vi "Alle Rohdaten abholen.vi"(7 "automatisch":bool, 8 "error in (no error)":errorcluster caption="Fehler (Eingang, kein Fehler)", 10 "Temp. Messzelle G-nr.":i32, 11 "Gasindex":i32) -> (0 "error out":errorcluster caption="Fehler (Ausgang)", 3 "Gasindex out":i32)   [LabVIEW 2020, in "Linearisierung v2.lvlib"]
uses:
  Linearisierung v2.lvlib
  Messdaten/Aktionen FGV Messdaten.ctl
  Aktion FGV Rohmesswerte sammeln.ctl
  Seiten/FT-IR/Aktionen EVID-Codes.ctl
  Seiten/FT-IR/FGV FT-IR Aktionen.ctl
  Messdaten/Gewichtung (Stichprobe).ctl
  Messdaten/Messdaten.lvlib
  Seiten/FT-IR/FT-IR.lvlib
  Seiten/FT-IR/FGV FT-IR Gasliste Aktionen.ctl
  cRIO/PC/Kommunikation mit cRIO.lvlib
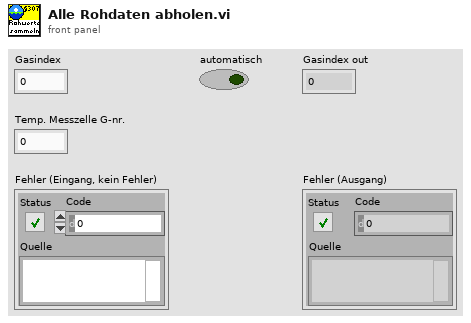
[diagram p1: front panel]
types:
  T1 = typedef "FT-IR.lvlib/FGV FT-IR Aktionen.ctl" = enum16{"lesen", "NOG setzen", "NOS setzen", "Initialisieren", "speichern", "ALLES setzen", "FT-IR Spektrum loggen", "Komm Stoppen", "Spektrum LogKonfig"}
  T2 = typedef "FT-IR.lvlib/Aktionen EVID-Codes.ctl" = enum16{"lesen", "setzen", "laden", "speichern", "1Hz/5Hz", "Smoothing", "Rolling Average"}
  T3 = typedef "Linearisierung v2.lvlib/Aktion FGV Rohmesswerte sammeln.ctl" = enum16{"lesen", "schreiben", "löschen", "Sollwert HovaCal"}
  T4 = typedef "Messdaten.lvlib/Aktionen FGV Messdaten.ctl" = enum16{"lesen", "schreiben", "löschen", "Mittelwerte", "Komponente"}
  T5 = typedef "FT-IR.lvlib/FGV FT-IR Gasliste Aktionen.ctl" = enum16{"lesen", "Gasliste FT-IR", "Gasliste ausgelesen", "laden", "speichern", "löschen"}
  T6 = typedef "String - Ausgabefeld.ctl" = string
  T7 = typedef "FT-IR.lvlib/1Hz-5Hz Geraet.ctl" = u16
  T8 = typedef "Verwaltung - cRIO.lvlib/Analog Eingaenge.ctl" = cluster{"AI0: Durchfluss FT-IR":sgl, "AI1: Druck Ausgang":sgl, "AI2: Umgebungsdruck":sgl, "AI3: Druck FT-IR":sgl, "AI4: Druck CalGas":sgl, "AI5: Reserve":sgl, "AI6: Reserve":sgl, "AI7: Reserve":sgl, "Rohwert Durchfluss FT-IR":sgl, "Rohwert Druck Ausgang":sgl, "Rohwert Umgebungsdruck":sgl, "Rohwert Druck FT-IR":sgl, "Rohwert Druck CalGas":sgl, "Rohwert AI5":sgl, "Rohwert AI6":sgl, "Rohwert AI7":sgl, "Rohwert Diffdruck mbar FTIR":sgl}
  T9 = cluster{"Aktuelle Messwert":dbl, "Aktuelle Rohwert":dbl, "Deviation":dbl, "Temp":dbl, "Druck":dbl, "Druchfluss":dbl}
  T10 = typedef "Messdaten.lvlib/Gewichtung (Stichprobe).ctl" = enum16{"Sample", "Population"}
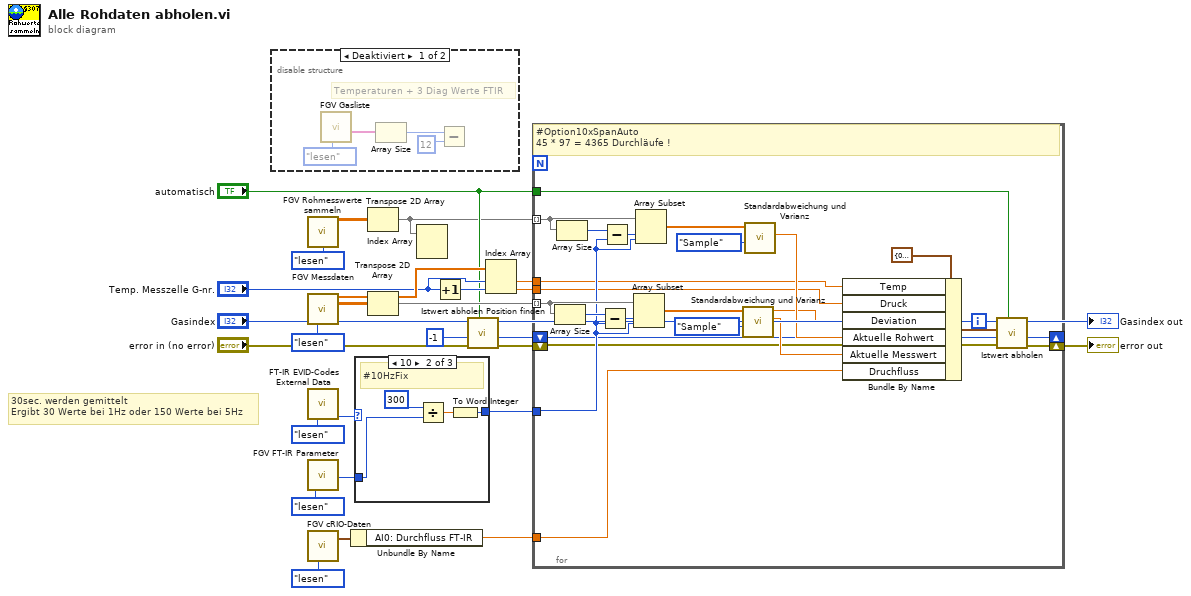
[diagram p0: block diagram]
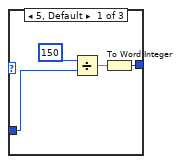
[diagram p3: hidden frame]
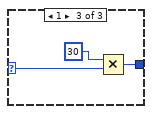
[diagram p4: hidden frame]
diagram:
  # "30sec. werden gemittelt\nErgibt 30 Werte bei 1Hz oder 150 Werte bei 5Hz"
  n1 = disable-structure shown="Deaktiviert" {
    frame Disabled {
      # "Temperaturen + 3 Diag Werte FTIR"
      n2 = call "FGV Gasliste.vi"("Aktionen"=FGV_FT-IR_Gasliste_Aktionen."lesen") -> ("Aktuelle Gasliste gesamt"=w28:T6[])  [unwired: 8 in, 2 out]
      n3 = Array Size(array=w28) -> (size(s)=w30:i32)
      n4 = Subtract(x=w30, y=12) -> ()  [unwired: 1 out]
    }
    frame Enabled {
    }
  }
  n5 = call "FGV Rohmesswerte sammeln.vi"("Aktion"=Aktion_FGV_Rohmesswerte_sammeln."lesen") -> ("Rohmessdaten"=w19:sgl[][])  [unwired: 11 in, 3 out]
  n6 = call "FGV Messdaten.vi"("Aktionen"=Aktionen_FGV_Messdaten."lesen") -> ("Aktuelle Messwerte"=w12:sgl[], "Messdaten"=w26:sgl[][])  [unwired: 6 in, 7 out]
  n7 = call "FT-IR EVID-Codes External Data.vi"("Aktionen"=Aktionen_EVID-Codes."lesen") -> ("1Hz/5Hz Gerät"=w22:T7)  [unwired: 9 in, 5 out]
  n8 = call "FGV FT-IR Parameter.vi"("Aktion"=FGV_FT-IR_Aktionen."lesen") -> ("NoOfScan"=w21:u32)  [unwired: 11 in, 7 out]
  n9 = call "FGV cRIO-Daten.vi"("Aktion"=enum16{"lesen", "schreiben"}."lesen") -> ("Analog Input"=w16:T8)  [unwired: 9 in, 9 out]
  n10 = Unbundle By Name(w16) -> ("AI0: Durchfluss FT-IR"=w15:sgl)
  n11 = case shown="10" w22 {
    selector: w22 -> [_ _ w40]
    tunnel: [w32 w36 w41] -> w20
    tunnel: w21 -> [w34 w38 _]
    frame 5, Default {
      n12 = Divide(x=150, y=w34) -> (x/y=w33:dbl)
      n13 = To Word Integer(number=w33) -> (16bit integer=w32:i16)
    }
    frame 10 {
      # "#10HzFix"
      n14 = Divide(x=300, y=w38) -> (x/y=w37:dbl)
      n15 = To Word Integer(number=w37) -> (16bit integer=w36:i16)
    }
    frame 1 {
      n16 = Multiply(x=30, y=w40) -> (x*y=w41:i32)
    }
  }
  n17 = Transpose 2D Array(2D array=w19) -> (transposed array=w3:sgl[][])
  n18 = Transpose 2D Array(2D array=w26) -> (transposed array=w18:sgl[][])
  n19 = Index Array(array=w3) -> ()  [unwired: 2 in, 1 out]
  n20 = Increment(x="Temp. Messzelle G-nr.") -> (x+1=w13:i32)
  n21 = call "Istwert abholen Position finden.vi"("automatisch"="automatisch", "error in (no error)"="error in (no error)", "Position Index in"=-1 ("Position Index out"), "Gasindex"="Gasindex") -> ("error out"=w7:errorcluster, "Position Index out"=w6:i32, "Gasindex out"=→"Gasindex out":i32)  [unwired: 5 in]
  n22 = Index Array(array=w12, index #1="Temp. Messzelle G-nr.", index #2=w13) -> (element #1=w10:sgl, element #2=w9:sgl)
  n23 = for {
    tunnel: w18 -> [w65] mode=indexing
    tunnel: w20 -> [w57]
    tunnel: w3 -> [w54] mode=indexing
    tunnel: w15 -> [w50]
    tunnel: "automatisch" -> [w49]
    shift-right: [w48] -> w14
    shift-left: w7 -> [w47]
    tunnel: w10 -> [w46]
    tunnel: w9 -> [w45]
    shift-right: [w44] -> _
    shift-left: w6 -> [w43]
    i -> [w53]
    # "#Option10xSpanAuto\n45 * 97 = 4365 Durchläufe !"
    n24 = Array Size(array=w65) -> (size(s)=w67:i32)
    n25 = Array Size(array=w54) -> (size(s)=w58:i32)
    n26 = Subtract(x=w67, y=w57) -> (x-y=w66:i32)
    n27 = Subtract(x=w58, y=w57) -> (x-y=w59:i32)
    n28 = Array Subset(array=w65, index=w66, length=w57) -> (w63:sgl[])
    n29 = Array Subset(array=w54, index=w59, length=w57) -> (w61:sgl[])
    n30 = call "Standardabweichung und Varianz.vi"("Gewichtung (Stichprobe)"=Gewichtung_(Stichprobe)."Sample", "X"=w63) -> ("Mittelwert"=w62:sgl, "Standardabweichung"=w55:sgl)  [unwired: 7 in, 1 out]
    n31 = call "Standardabweichung und Varianz.vi"("Gewichtung (Stichprobe)"=Gewichtung_(Stichprobe)."Sample", "X"=w61) -> ("Mittelwert"=w56:sgl)  [unwired: 7 in, 2 out]
    n32 = Bundle By Name(cluster=T9 {"Aktuelle Messwert"=0.0, "Aktuelle Rohwert"=0.0, "Deviation"=0.0, "Temp"=0.0, "Druck"=0.0, "Druchfluss"=0.0} ("Eingangswerte"), "Temp"=w46, "Druck"=w45, "Deviation"=w55, "Aktuelle Rohwert"=w56, "Aktuelle Messwert"=w62, "Druchfluss"=w50) -> (w51:T9)
    n33 = call "Istwert abholen.vi"("automatisch"=w49, "error in (no error)"=w47, "Position Index in"=w43, "Eingangswerte"=w51, "Gasindex"=w53) -> ("error out"=w48:errorcluster, "Position Index out"=w44:i32)  [unwired: 5 in]
  }
  "error out" <- w14
